vi "Fetch Multiple Record Multiple Channel (DBL).vi"(5 "FIFO Type":enum16{"FPGA to Host FIFO (U64)", "Generic"}(ring), 7 "Timeout (s)":i32=5, 8 "error in":errorcluster, 10 "Records to Fetch":i32, 11 "FPGA VI Reference In":refnum<k20>) -> (0 "error out":errorcluster, 2 "Acquired Data":dbl[][](array[numeric]) format="%.2f", 3 "FPGA VI Reference Out":refnum<k20>, 4 "Elements Remaining":u32)   [LabVIEW 2011]
uses:
  <userlib>/FlexRIO Host Library/FlexRIO Host API/Acquire/Fetch/Fetch Acquired Data (U64).vi
  <vilib>/Utility/error.llb/Error Cluster From Error Code.vi
  <vilib>/rvi/errors/niLvFpgaAdjustHostInterfaceError.vi
  <vilib>/rvi/interface/nirviReadWriteControl/nirviReadWriteControl.xnode
  NiFpgaLv.dll
  <vilib>/rvi/interface/Simulation/niFpgaSimulationCallBeginRW.vi
  <userlib>/FlexRIO Host Library/FlexRIO Host Library (User).lvlib
  <userlib>/FlexRIO Host Library/FlexRIO Host API/Utility/memnoncopy.dll
panel:
  out "Data Acquired":i16[](array[numeric])
  out "Dummy Data":i16[](array[numeric])
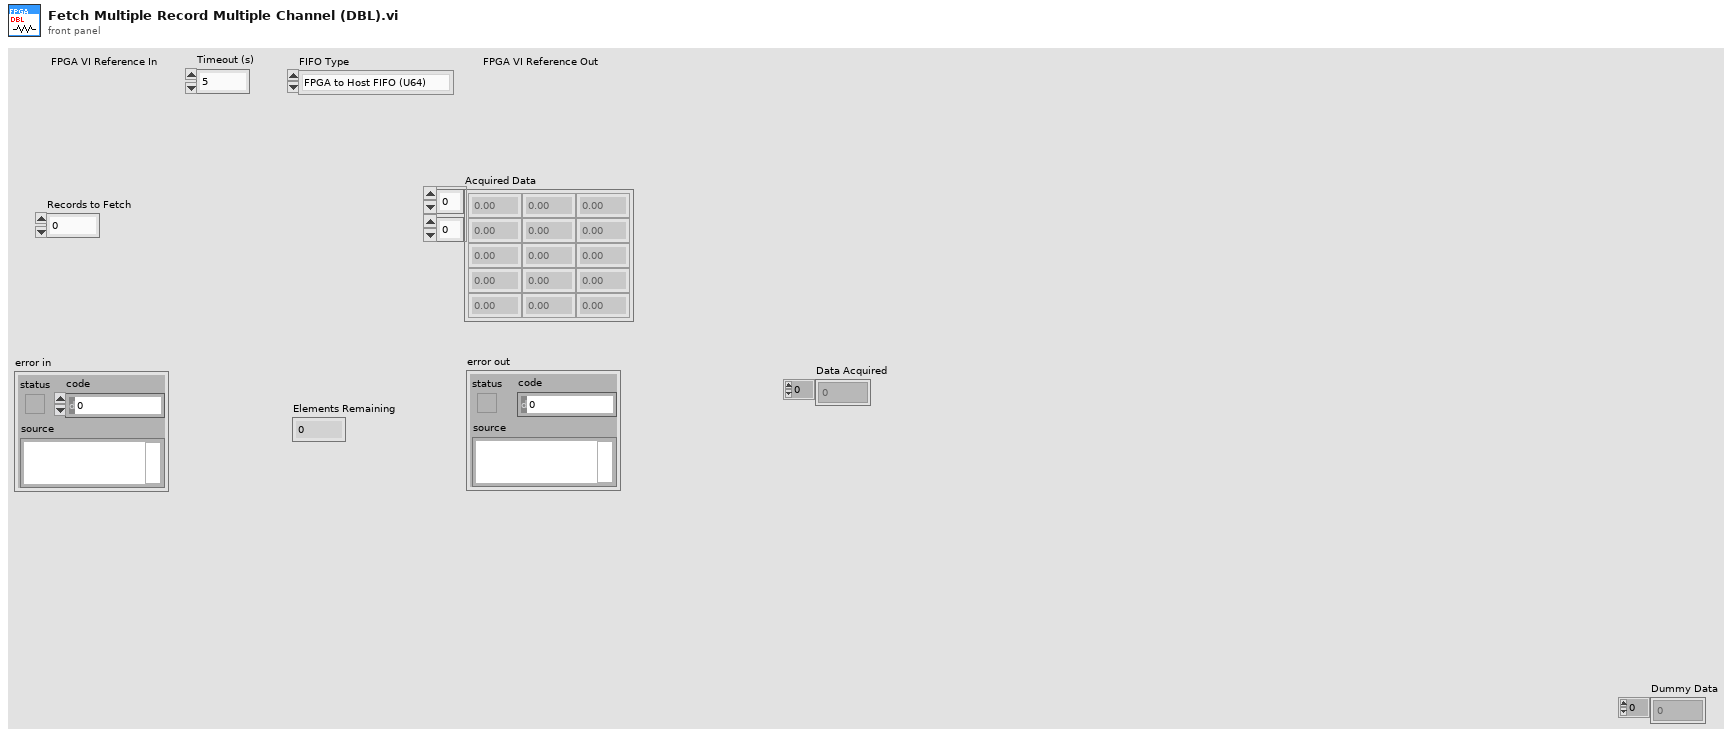
[diagram p1: front panel]
types:
  T1 = cluster{"Load Record Parameters?":bool, "Pre Trigger Samples":u16, "Samples per Record":u16, "Trigger Hold Off":u16, "Record Count":u16}
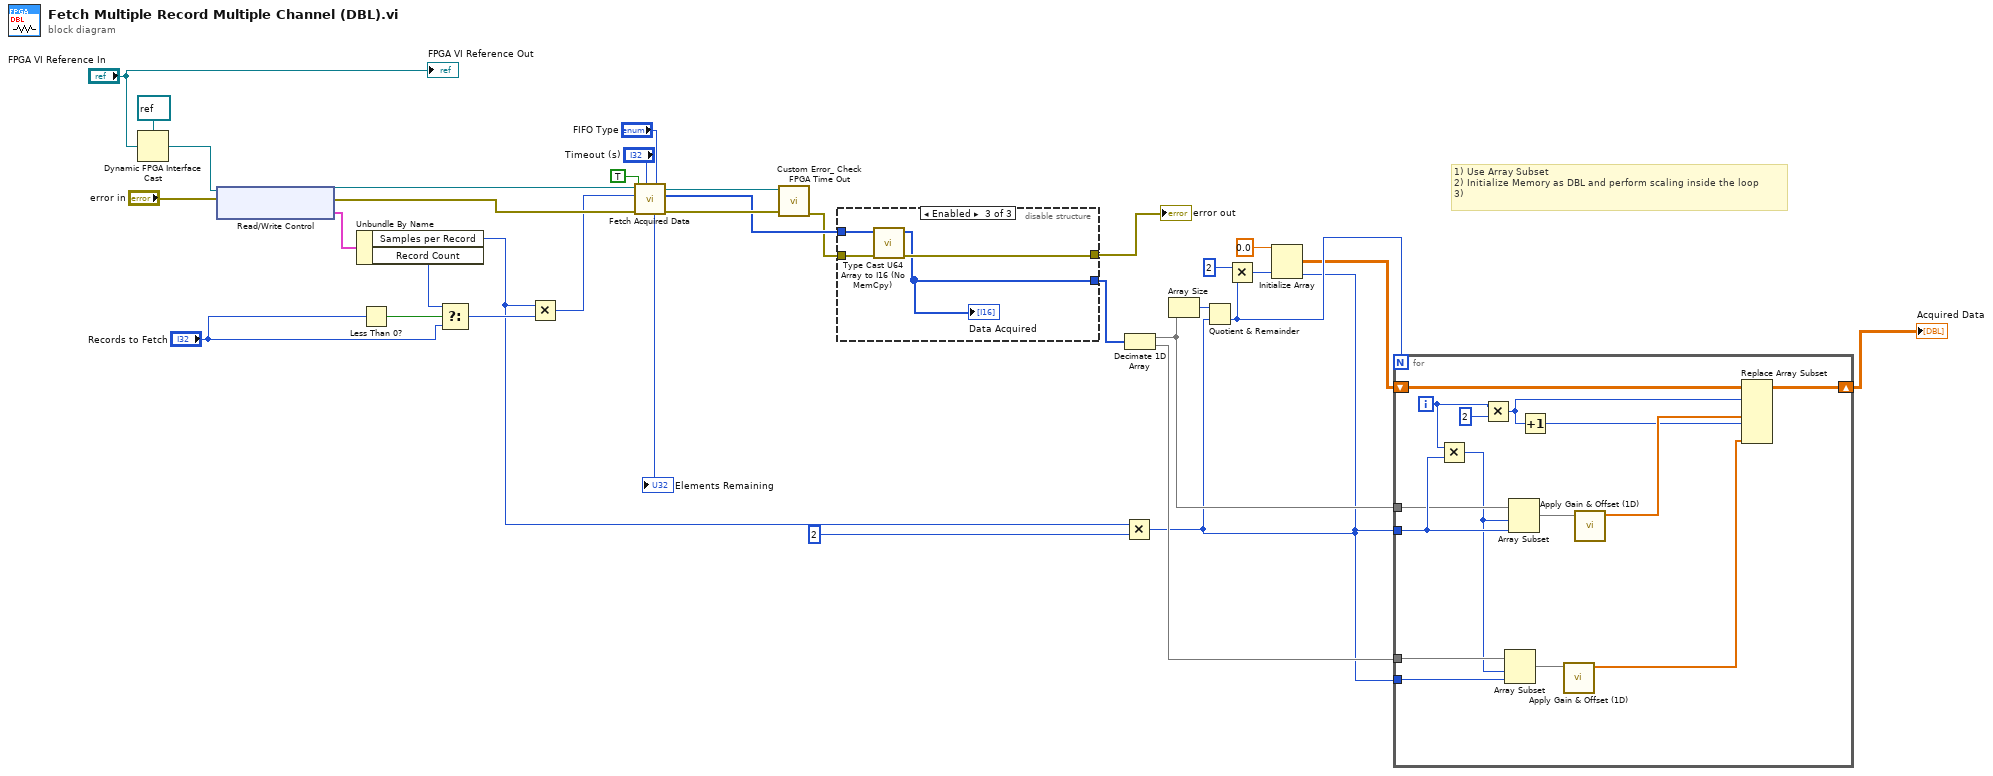
[diagram p0: block diagram]
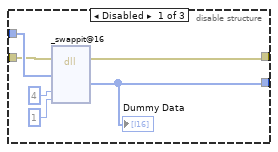
[diagram p2: hidden frame]
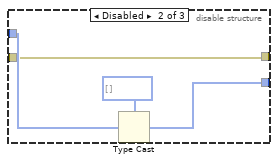
[diagram p3: hidden frame]
diagram:
  # "1) Use Array Subset\n2) Initialize Memory as DBL and perform scaling inside the loop\n3)"
  n1 = Dynamic FPGA Interface Cast(Session In=refnum<k20> refnum ("Type"), Type="FPGA VI Reference In") -> (Session Out=w31:refnum<k20>)
  n2 = xnode "Read/Write Control"("FPGA VI Reference In"=w31, "error in"="error in") -> ("FPGA VI Reference Out"=w26:refnum<k20>, "error out"=w25:errorcluster, "Record Parameters"=w30:T1)
  n3 = Unbundle By Name(w30) -> ("Samples per Record"=w19:u16, "Record Count"=w28:u16)
  n4 = Less Than 0?(x="Records to Fetch") -> (x < 0?=w29:bool)
  n5 = Select(t=w28, s=w29, f="Records to Fetch") -> (s? t:f=w20:i32)
  n6 = Multiply(x=w19, y=w20) -> (x*y=w24:i32)
  n7 = call-poly <userlib>:"Fetch Acquired Data.vi"("FIFO Type"="FIFO Type", "Timeout (s)"="Timeout (s)", "error out"=w25, "Swap?"=TRUE, "Samples"=w24, "FPGA Reference In"=w26) -> ("error out"=w14:errorcluster, "Data"=w5:u64[], "FPGA Reference Out"=w15:refnum<k20>, "Elements Remaining"=→"Elements Remaining":u32)  [unwired: 2 in]
  n8 = call <userlib>:"Custom Error_ Check FPGA Time Out.vi"("error in"=w14, "FPGA VI Reference In"=w15) -> ("error out"=w4:errorcluster)  [unwired: 8 in, 1 out]
  n9 = disable-structure shown="Enabled" {
    disable-tunnel: w5 -> [w38 w43 w48]
    disable-tunnel: w4 -> [w37 w41 w47]
    disable-tunnel: [w36 w41 w46] -> w3
    disable-tunnel: [w35 w42 w45] -> w2
    frame Disabled {
      n10 = dll-call lib="C:/Program Files (x86)/National Instruments/LabVIEW 2011/user.lib/FlexRIO Host Library/FlexRIO Host API/Utility/memnoncopy.dll" fn="_swappit@16"(error in=w37, "src"=w38, "upsize"=4, "downsize"=1) -> (error out=w36:errorcluster, "Dummy Data"=w35:i16[])  [unwired: 7 in, 1 out]
      "Dummy Data" <- w35
    }
    frame Disabled {
      n11 = Type Cast(type=i16[] [], x=w43) -> (*(type *) &x=w42:i16[])
    }
    frame Enabled {
      n12 = call <userlib>:"Type Cast U64 Array to I16 (No MemCpy).vi"("error in"=w47, "Input"=w48) -> ("error out"=w46:errorcluster, "Data Acquired"=w45:i16[])  [unwired: 8 in]
      "Data Acquired" <- w45
    }
  }
  "error out" <- w3
  n13 = Multiply(x=w19, y=u16 2) -> (x*y=w7:u16)
  n14 = Decimate 1D Array(w2) -> (w17:i16[], w8:i16[])
  n15 = Array Size(array=w17) -> (size(s)=w16:i32)
  n16 = Quotient & Remainder(x=w16, y=w7) -> (floor(x/y)=w11:i32)  [unwired: 1 out]
  n17 = Multiply(x=2, y=w11) -> (x*y=w12:i32)
  n18 = Initialize Array(0.0 ("element"), w12, w7) -> (w9:dbl[][])
  n19 = for {
    N: w11 -> [_]
    tunnel: w17 -> [w62]
    tunnel: w7 -> [w63]
    tunnel: w8 -> [w61]
    tunnel: w7 -> [w59]
    shift-right: [w57] -> w6
    shift-left: w9 -> [w58]
    i -> [w54]
    n20 = Multiply(x=w54, y=w63) -> (x*y=w60:i32)
    n21 = Multiply(x=w54, y=2) -> (x*y=w52:i32)
    n22 = Array Subset(array=w61, index=w60, length=w59) -> (w55:i16[])
    n23 = Array Subset(array=w62, index=w60, length=w63) -> (w56:i16[])
    n24 = Increment(x=w52) -> (x+1=w50:i32)
    n25 = call <userlib>:"Apply Gain & Offset (1D).vi"("Raw Data"=w55) -> ("Scaled Data"=w49:dbl[])  [unwired: 10 in]
    n26 = call <userlib>:"Apply Gain & Offset (1D).vi"("Raw Data"=w56) -> ("Scaled Data"=w51:dbl[])  [unwired: 10 in]
    n27 = Replace Array Subset(array=w58, new element #1=w51, index (row) #1=w52, new element #2=w49, index (row) #2=w50) -> (w57:dbl[][])  [unwired: 2 in]
  }
  "Acquired Data" <- w6
  "FPGA VI Reference Out" <- "FPGA VI Reference In"
